vi "Write JSON Config.vi"(6 "Pretty Print?":bool, 8 "error in (no error)":errorcluster, 11 "Const_U64 in":refnum<class "Const_U64.lvclass">) -> (0 "error out":errorcluster, 2 "JSON":string, 3 "Const_U64 out":refnum<class "Const_U64.lvclass">)   [LabVIEW 2021, in "Const_U64.lvclass"]
uses:
  Const_U64.lvclass
  C:/Program Files (x86)/National Instruments/LabVIEW 2021/vi.lib/TSA/Abstract Data Classes/Abs_Types/Type/Abs_Type.lvclass
  Const_U64.lvclass/Const_U64.ctl
  e5c4abb0-945c-4713-8383-6c7088636957.vi
  <vilib>/Utility/LVClass/Get LV Class Name.vi
  <vilib>/JDP Science/JSONtext/Variant to JSON Text.vi
  <vilib>/JDP Science/JSONtext/Set Multiple Object Items.vi
  <vilib>/JDP Science/JSONtext/LVClass Serializer/JSONtext LVClass Serializer.lvclass
  Abs_Types/U64 Integer/Abs_U64 Integer.lvclass
  Abs_Types/Type/Abs_Type.lvclass
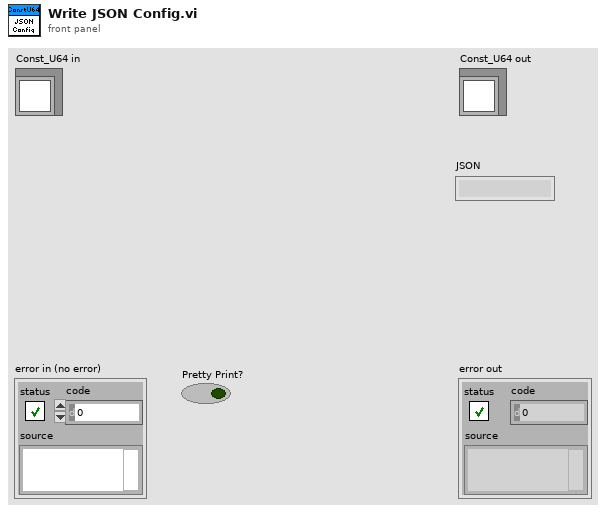
[diagram p1: front panel]
types:
  T1 = typedef "Const_U64.lvclass/Type.ctl" = u64
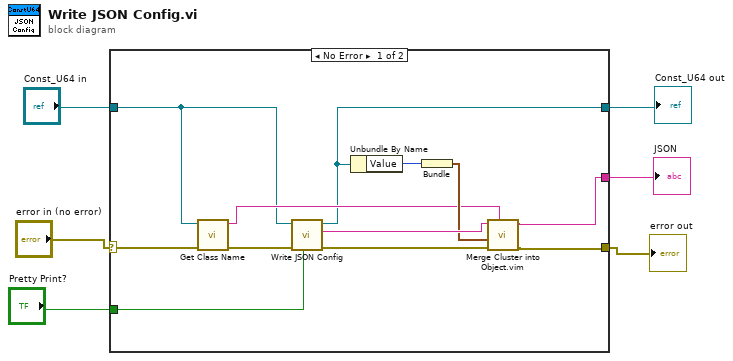
[diagram p0: block diagram]
diagram:
  n1 = case shown="No Error" "error in (no error)" {
    selector: "error in (no error)" -> [w17 w20]
    tunnel: [w11 w20] -> w6
    tunnel: [w12 _] -> w2
    tunnel: [w8 w19] -> w1
    tunnel: "Const_U64 in" -> [w10 w19]
    tunnel: "Pretty Print?" -> [w7 _]
    frame No Error {
      n2 = call "Get Class Name.vi"("error in (no error)"=w17, "Abs_Type in"=w10) -> ("error out"=w18:errorcluster, "class name"=w13:string)  [unwired: 8 in]
      n3 = call-parent "Write JSON Config.vi"("Pretty Print?"=w7, "error in (no error)"=w18, "Abs_Type in"=w10) -> ("error out"=w16:errorcluster, "JSON"=w15:string, "Abs_Type out"=w8:refnum<class "Const_U64.lvclass">)  [unwired: 6 in]
      n4 = Unbundle By Name(w8) -> ("Value"=w9:T1)
      n5 = Bundle("Value"=w9) -> (w14:cluster{"Value":T1})  [unwired: 1 in]
      n6 = call "Merge Cluster into Object.vim"("$Path or Item Name"=w13, "error in (no error)"=w16, "Any Cluster"=w14, "JSON"=w15) -> ("error out"=w11:errorcluster, "<JSON>"=w12:string)  [unwired: 5 in]
    }
    frame Error {
    }
  }
  "error out" <- w6
  "Const_U64 out" <- w1
  "JSON" <- w2
